vi "Get UC tick taus.vi"(2 "Log Tick Start (-10: 100 ps)":i32=-10, 3 "# Decades (4: 10 ps - 900 ns)":i32=4) -> (7 "Array of taus":dbl[unit][](array[numeric]))   [LabVIEW 2019]
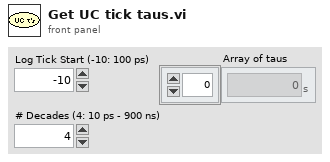
[diagram p1: front panel]
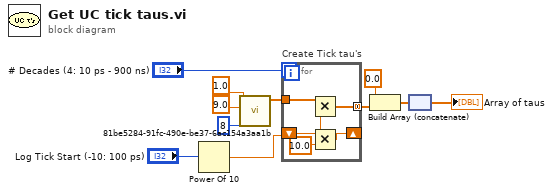
[diagram p0: block diagram]
diagram:
  n1 = Power Of 10(x="Log Tick Start (-10: 100 ps)") -> (10^x=w3:dbl)
  n2 = call "81be5284-91fc-490e-be37-6ac154a3aa1b.vi"("# Steps (1)"=8, "End (1)"=9.0 ("Start (0)"), "Start (0)"=1.0 ("End (1)")) -> ("Ramp"=w4:dbl[])  [unwired: 7 in, 1 out]
  n3 = for "Create Tick tau's" {
    N: "# Decades (4: 10 ps - 900 ns)" -> [_]
    shift-right: [w15] -> _
    shift-left: w3 -> [w14]
    tunnel: w4 -> [w13]
    tunnel: [w12] -> w5 mode=concatenating
    n4 = Multiply(x=w13, y=w14) -> (x*y=w12:dbl[])
    n5 = Multiply(x=w14, y=10.0) -> (x*y=w15:dbl)
  }
  n6 = Build Array (concatenate)(0.0 ("End (1)"), w5) -> (w10:dbl[])
  n7 = node(w10) -> (→"Array of taus":dbl[unit][])
